vi "Const Strings.vi"() -> ()   [LabVIEW 2017, in "WebServiceImporter.lvlib"]
uses:
  <vilib>/Platform/WebService/WebServiceImporter.lvlib
panel:
  in  "Creating Menu File...":string="Creating Menu File..."
  in  "Msg for Project Library or VI already in memory":string="The destination project or library or VIs that will be generated during the process are already opened in the memory. \n\nPlease close them first or try changing either the library name or directory name."
  in  "File name warning":string="A library name cannot contain any of the following characters:\n\\ / : * ? \" < > |"
  in  "WSDL Incorrect Message":string="SOAP protocol is not detected. We only support service using SOAP."
  in  "refnum out Label":string=" refnum out"
  in  "refnum Label":string=" refnum"
  in  "Import Failed":string="An error has occured while attempting to import the specified web service. Please check the report for detailed information."
  in  "Import Success":string="Web Service successfully imported."
  in  "Next Bool Text":string="Next"
  in  "Generate Bool Text":string="Generate"
  in  "Report error title":string="The following errors/warnings occurred when generating the local proxy dll and VI wrappers for this web service."
  in  "Report general title":string=".NET Web Service Proxy Tool Report for Web Service:"
  in  "No Error":string="There is no error."
  in  "Creating Wrapper VIs...":string="Creating Wrapper VIs..."
  in  "Creating Proxy Dll...":string="Creating Local Proxy DLL..."
  in  "Imported Data Types":string="Imported Data Types"
  in  "Imported Methods":string="Imported Methods"
  in  "Location":string="Location"
  in  "Library Name":string="Library Name"
  in  "Web Service Name":string="Web Service Name"
  in  "Web Service URL":string="Web Service URL"
  in  "Msg for Proxy Dll Existance":string="The project library already exists. Do you want to overwrite it? "
  in  "Skip":string="Cancel"
  in  "Overwrite":string="Overwrite"
  in  "Cancel Bool Text":string="Cancel"
  in  "Finish Bool Text":string="Finish"
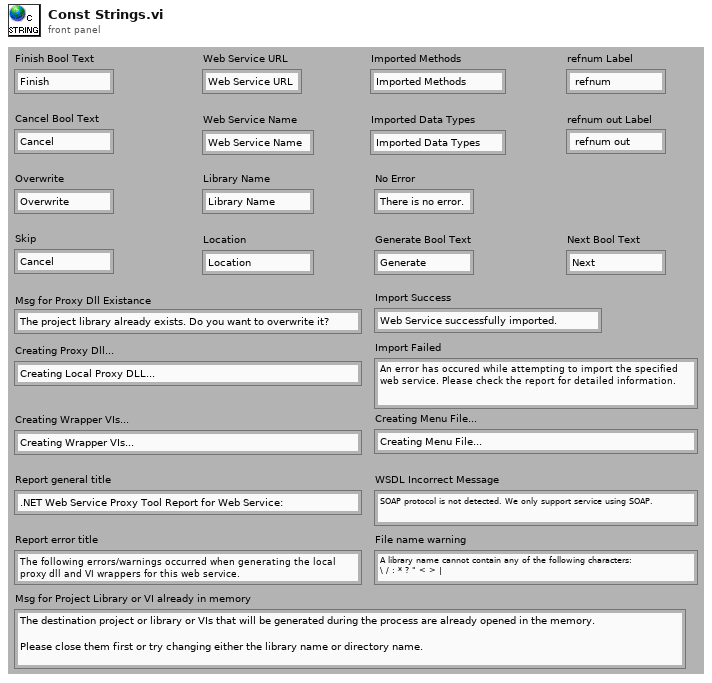
[diagram p1: front panel]
diagram:
